vi "osciloscopio.vi"() -> ()   [LabVIEW 2010]
uses:
  <vilib>/Utility/error.llb/DialogType.ctl
  <vilib>/express/express arith-compare/Formula/XNode/ExpressFormulaBlockNode.xnode
  <vilib>/DAQmx/read.llb/DAQmx Read.vi
  <vilib>/DAQmx/read.llb/DAQmx Read (Analog Wfm 1Chan NSamp).vi
  <vilib>/DAQmx/create/channels.llb/DAQmx Create Channel (AI-Voltage-Basic).vi
  <vilib>/DAQmx/configure/timing.llb/DAQmx Timing (Sample Clock).vi
  <vilib>/DAQmx/configure/trigger.llb/DAQmx Start Trigger (Digital Edge).vi
  <vilib>/daqmx/miscellaneous.llb/DAQmx Fill In Error Info.vi
  <vilib>/express/express shared/transition.llb/Dynamic To Waveform Array.vi
  <vilib>/express/express shared/transition.llb/Waveform Array To Dynamic.vi
  <vilib>/express/express arith-compare/Formula/Block/exnFormulaBlock how many pts in the wave.vi
  <vilib>/express/express shared/ex_Modify Signal Name.vi
panel:
  out "Trigger delay":dbl format="%#_6e"
  out "Signal":waveform(dbl)[](graph)
  in  "stop 2":bool
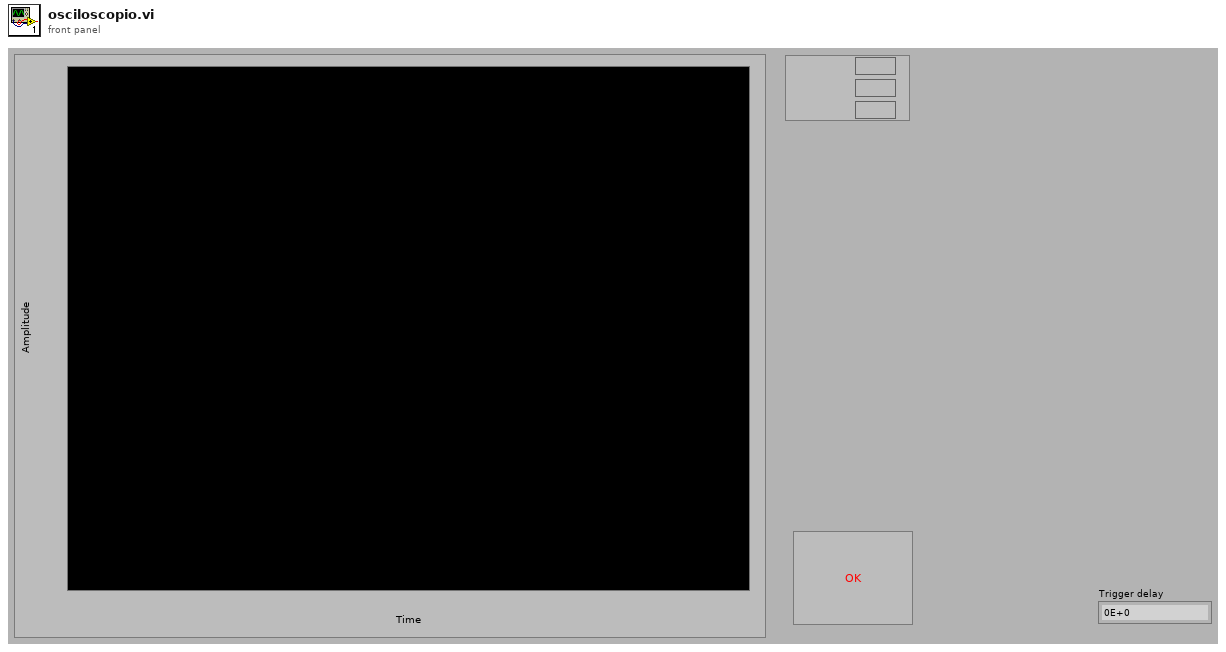
[diagram p1: front panel]
types:
  T1 = typedef "DialogType.ctl" = u16
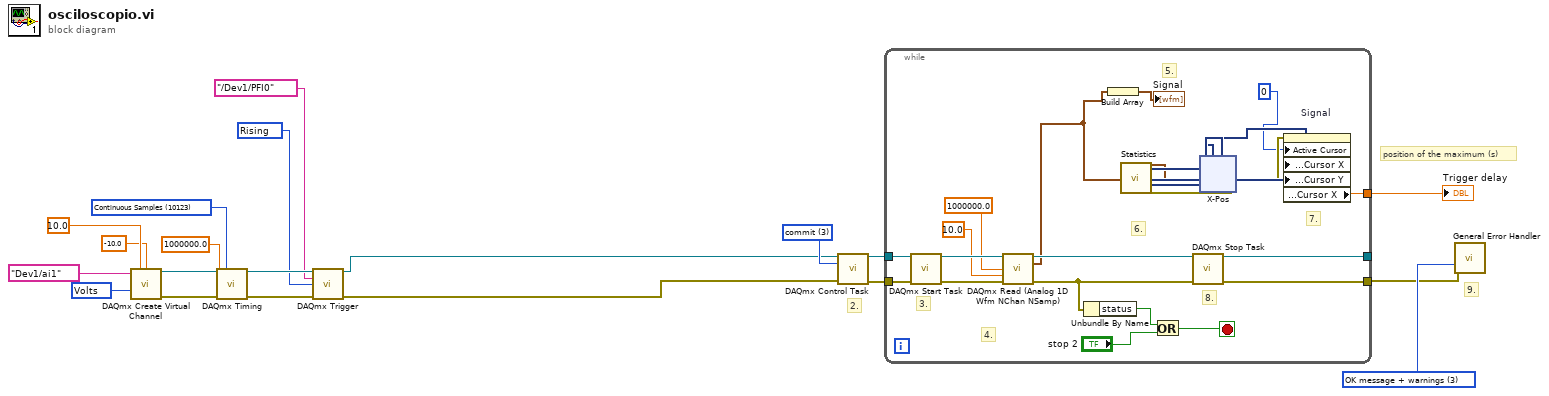
[diagram p0: block diagram]
diagram:
  w7 = T1 3 items=["no dialog", "OK message", "continue or stop message", "OK message + warnings", "continue/stop + warnings"] ("type of dialog (OK msg:1)")
  w8 = 3 items=["verify"=2, "reserve"=4, "commit"=3, "unreserve"=5, "abort"=6] ("action")
  w11 = 10280 items=["Rising"=10280, "Falling"=10171] ("edge")
  w13 = 10123 items=["Finite Samples"=10178, "Continuous Samples"=10123, "Hardware Timed Single Point"=12522] ("sample mode")
  w17 = 10348 items=["Volts"=10348, "From Custom Scale"=10065] ("units")
  # "position of the maximum (s)"
  # "9."
  # "2."
  n1 = call-poly <vilib>:"DAQmx Create Virtual Channel.vi"("maximum value"=10.0, "minimum value"=-10.0, "physical channels"=tag "Dev1/ai1", "units"=w17) -> ("task out"=w16:refnum<k21>, "error out"=w3:errorcluster)  [unwired: 10 in]
  n2 = call-poly <vilib>:"DAQmx Timing.vi"("task/channels in"=w16, "sample mode"=w13, "rate"=1000000.0, "error in"=w3) -> ("task out"=w15:refnum<k21>, "error out"=w4:errorcluster)  [unwired: 10 in]
  n3 = call-poly <vilib>:"DAQmx Trigger.vi"("task/channels in"=w15, "source"=tag "/Dev1/PFI0", "edge"=w11, "error in"=w4) -> ("task out"=w2:refnum<k21>, "error out"=w1:errorcluster)  [unwired: 10 in]
  n4 = call <vilib>:"DAQmx Control Task.vi"("task/channels in"=w2, "action"=w8, "error in"=w1) -> ("task out"=w10:refnum<k21>, "error out"=w9:errorcluster)  [unwired: 11 in]
  n5 = while {
    tunnel: w10 -> [w43]
    tunnel: w9 -> [w42]
    tunnel: [w41] -> w5
    tunnel: [w28] -> _
    tunnel: [w27] -> w6
    stop <- w23 stop-if-true
    # "8."
    # "6."
    # "7."
    # "5."
    # "4."
    # "3."
    n6 = call <vilib>:"DAQmx Start Task.vi"("task/channels in"=w43, "error in"=w42) -> ("task out"=w40:refnum<k21>, "error out"=w39:errorcluster)  [unwired: 12 in]
    n7 = call-poly "DAQmx Read (Analog 1D Wfm NChan NSamp).vi"("task/channels in"=w40, "number of samples per channel"=1000000.0 ("Samples/channel"), "timeout"=10.0, "error in"=w39) -> ("task out"=w38:refnum<k21>, "data"=w21:waveform(dbl), "error out"=w25:errorcluster)  [unwired: 9 in]
    n8 = Unbundle By Name(w25) -> ("status"=w26:bool)
    n9 = Build Array(w21) -> (→"Signal":waveform(dbl)[])
    n10 = call "Statistics"("Signals"=w21) -> ("First Time"=w34:dynamicdata, "Time of Maximum"=w35:dynamicdata, "Maximum"=w33:dynamicdata, "error out"=w32:errorcluster)  [unwired: 21 in, 2 out]
    n11 = Or(x=w26, y="stop 2") -> (x .or. y?=w23:bool)
    n12 = call <vilib>:"DAQmx Stop Task.vi"("task/channels in"=w38, "error in"=w25) -> ("task out"=w28:refnum<k21>, "error out"=w27:errorcluster)  [unwired: 12 in]
    n13 = xnode "X-Pos"("TimeMax"=w35, "1stTime"=w34, "error in (no error)"=w32) -> ("Result"=w29:dynamicdata, "error out"=w31:errorcluster)
    n14 = property on="Signal" class="WFGraph (strict)"(error in=w31, "Active Cursor"=u32 0, "Cursor.Cursor Position:Cursor X"=w29, "Cursor.Cursor Position:Cursor Y"=w33) -> ("Cursor.Cursor Position:Cursor X"=w41:dbl)  [unwired: 1 in, 2 out]
  }
  "Trigger delay" <- w5
  n15 = call <vilib>:"General Error Handler.vi"("type of dialog (OK msg:1)"=w7, "error in (no error)"=w6) -> ()  [unwired: 9 in, 5 out]
